vi "save_data.vi"(5 "Array of ROI sums":dbl[][](array[numeric]), 7 "Current Measurement":u32, 8 "error in (no error)":errorcluster, 9 "ExperimentVariables (in)":refnum<class "ExperimentVariables.lvclass">, 10 "Counter (in)":refnum<class "Counter.lvclass">, 11 "Camera (in)":refnum<class "Hamamatsu_C9100-13.lvclass">) -> (0 "error out":errorcluster, 1 "ExperimentVariables":refnum<class "ExperimentVariables.lvclass">, 2 "Counter":refnum<class "Counter.lvclass">, 3 "Camera":refnum<class "Hamamatsu_C9100-13.lvclass">)   [LabVIEW 2013]
uses:
  ExperimentVariables/ExperimentVariables.lvclass
  Counter/Counter.lvclass
  Camera/Hamamatsu_C9100-13/Hamamatsu_C9100-13.lvclass
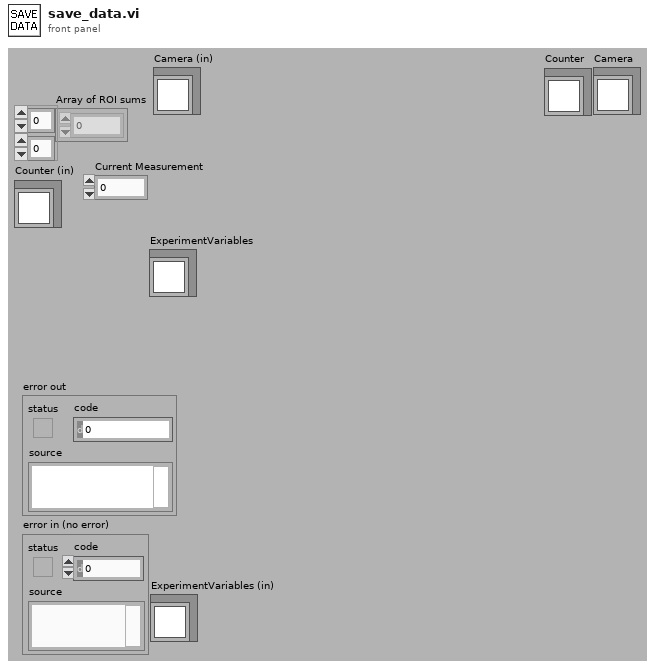
[diagram p1: front panel]
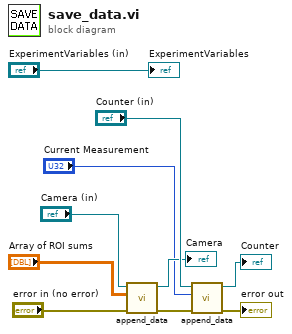
[diagram p0: block diagram]
diagram:
  n1 = call-dynamic "append_data.vi"("error in (no error)"="error in (no error)", "Array of ROI sums"="Array of ROI sums", "Camera in"="Camera (in)") -> ("error out"=w6:errorcluster, "Camera out"=→"Camera":refnum<class "Hamamatsu_C9100-13.lvclass">)  [unwired: 7 in]
  n2 = call-dynamic "append_data.vi"("error in (no error)"=w6, "Current measurement #"="Current Measurement", "Counter in"="Counter (in)") -> ("error out"=→"error out":errorcluster, "Counter out"=→"Counter":refnum<class "Counter.lvclass">)  [unwired: 7 in]
  "ExperimentVariables" <- "ExperimentVariables (in)"
